vi "rs3 get stream profiles.vi"(8 "error in (no error)":errorcluster, 11 "Sensor in":u64) -> (0 "error out":errorcluster, 1 "Stream profile list":u64, 2 "error out":u64, 3 "Sensor out":u64)   [LabVIEW 2017, in "libRealSense3.lvlib"]
doc: "Provides the Stream Profile List (handle) that should be used together with \"STREAM PROFILE\", \"STREAM PROFILE COUNT\" and \"STREAM PROFILE INFO\" to describe the selected SENSOR."
uses:
  libRealSense3.lvlib
  realsense2.dll
panel:
  # "RS3 Get Stream Profiles"
  # "(C) Intel Corp.,  AGJ 2017"
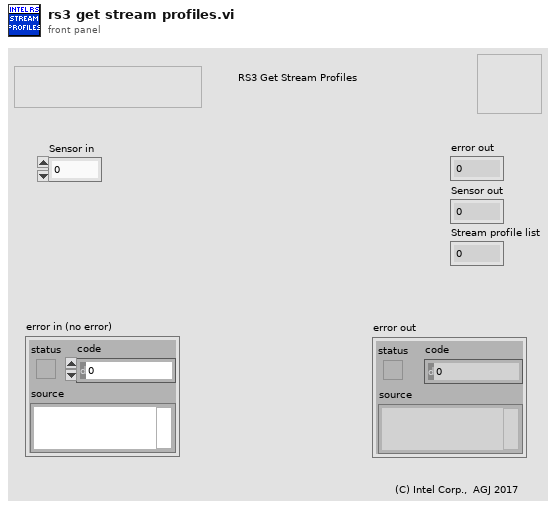
[diagram p1: front panel]
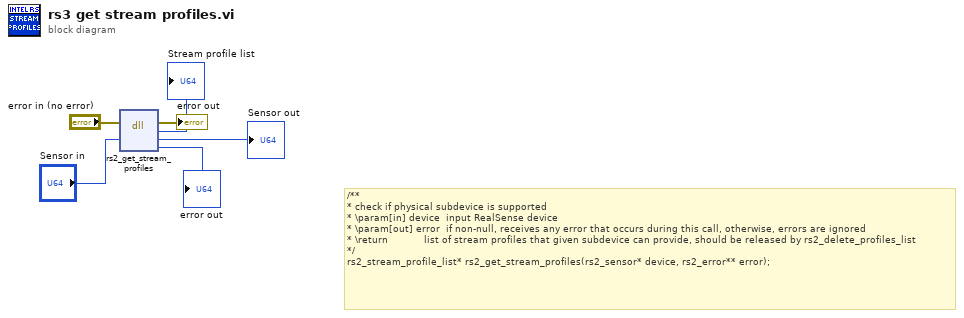
[diagram p0: block diagram]
diagram:
  # "/**\n* check if physical subdevice is supported\n* \\param[in] device  input RealSense device\n* \\param[out] error  if non-null, receives any error that occurs during this call, otherwise, errors are ignored\n* \\return            list of stream profiles that given subdevice can provide, should be released by rs2_delete_profiles_list\n*/\nrs2_stream_profile_list* rs2_get_stream_profiles(rs2_sensor* device, rs2_error** error);"
  n1 = dll-call lib="C:/Users/smartek/Desktop/labview/realsense2.dll" fn="rs2_get_stream_profiles"(error in="error in (no error)", "frame"="Sensor in") -> (error out=→"error out":errorcluster, "stream profile list"=→"Stream profile list":u64, "frame"=→"Sensor out":u64, "error"=→"error out":u64)  [unwired: 3 in, 1 out]
